vi "XYZStage-Initialisation.vi"(8 "Error In":errorcluster, 11 "XY Stage":T1) -> (0 "Error Out":errorcluster, 3 "VISA resource name out":refnum<visa-resource-name>)   [LabVIEW 2013]
uses:
  Typedefs/XY Stage config cluster.ctl
  Globals/gl_XYZStage globals.vi
  <vilib>/Instr/_visa.llb/VISA Configure Serial Port (Instr).vi
panel:
  in  "flow control":u16(ring) items=["None"=0, "XON/XOFF"=1, "RTS/CTS"=2, "DTR/DSR"=4]
  in  "stop bits":u16(ring)=10 items=["1.0"=10, "1.5"=15, "2.0"=20]
  in  "parity":u16(ring) items=["None", "Odd", "Even", "Mark", "Space"]
  in  "data bits":u16=8 min=5 max=8 step=1
  in  "baud rate":u32=9600
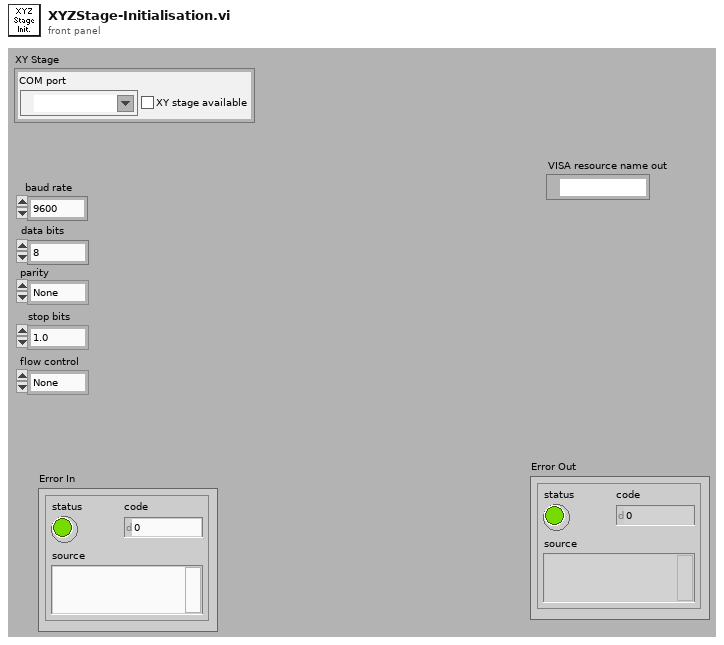
[diagram p1: front panel]
types:
  T1 = typedef "XY Stage config cluster.ctl" = cluster{"COM port":refnum<visa-resource-name>, "XY stage available":bool}
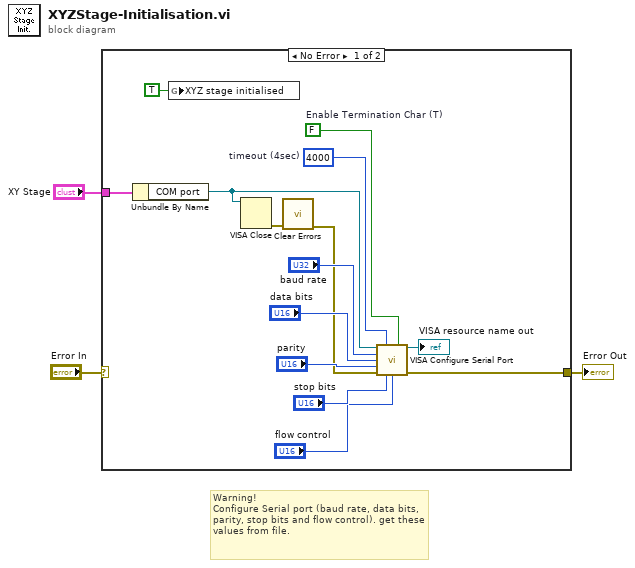
[diagram p0: block diagram]
diagram:
  # "Warning!\nConfigure Serial port (baud rate, data bits, parity, stop bits and flow control). get these values from file."
  n1 = case shown="No Error" "Error In" {
    selector: "Error In" -> [_ w18]
    tunnel: [w9 w18] -> w3
    tunnel: "XY Stage" -> [w8 _]
    frame No Error {
      w13 = FALSE  # Enable Termination Char (T)
      w14 = u32 4000  # timeout (4sec)
      n2 = Unbundle By Name(w8) -> ("COM port"=w7:refnum<visa-resource-name>)
      n3 = global write "gl_XYZStage globals.vi" "XYZ stage initialised"(TRUE ("XYZ stage initialised")) -> ()
      n4 = VISA Close(VISA resource name=w7) -> (error out=w6:errorcluster)  [unwired: 1 in]
      n5 = call <vilib>:"Clear Errors.vi"("error in (no error)"=w6) -> ("error out"=w5:errorcluster)  [unwired: 6 in]
      n6 = call-poly "VISA Configure Serial Port"("VISA resource name"=w7, "timeout (10sec)"=w14, "Enable Termination\nChar (T)"=w13, "baud rate (9600)"="baud rate", "data bits (8)"="data bits", "parity (0:none)"="parity", "error in (no error)"=w5, "stop bits (10: 1 bit)"="stop bits", "flow control (0:none)"="flow control") -> ("VISA resource name out"=→"VISA resource name out":refnum<visa-resource-name>, "error out"=w9:errorcluster)  [unwired: 5 out]
    }
    frame Error {
    }
  }
  "Error Out" <- w3
